vi "Grade_Saver.vi"() -> ()   [LabVIEW 2010]
panel:
  out "Letter Grade":string
  out "Final Grade":dbl
  out "Letter Grade":string
  out "Points":dbl
  in  "MP3":dbl
  out "Points":dbl
  out "Letter Grade":string
  in  "Exam":dbl
  out "Semester Grade":dbl
  out "Letter Grade":string
  out "Points":dbl
  out "Letter Grade":string
  in  "MP4":dbl
  out "Letter Grade":string
  out "Semester Grade":dbl
  out "Points":dbl
  out "Letter Grade":string
  in  "Exam":dbl
  out "Points":dbl
  out "Letter Grade":string
  in  "MP2":dbl
  out "Points":dbl
  out "Letter Grade":string
  in  "MP1":dbl
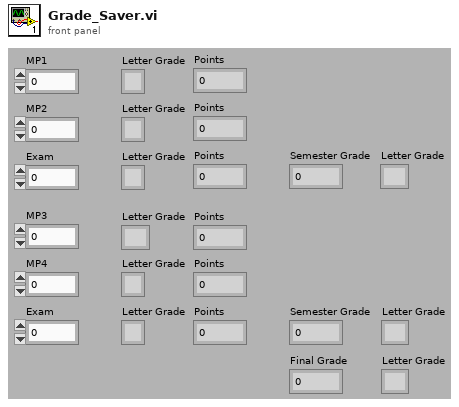
[diagram p1: front panel]
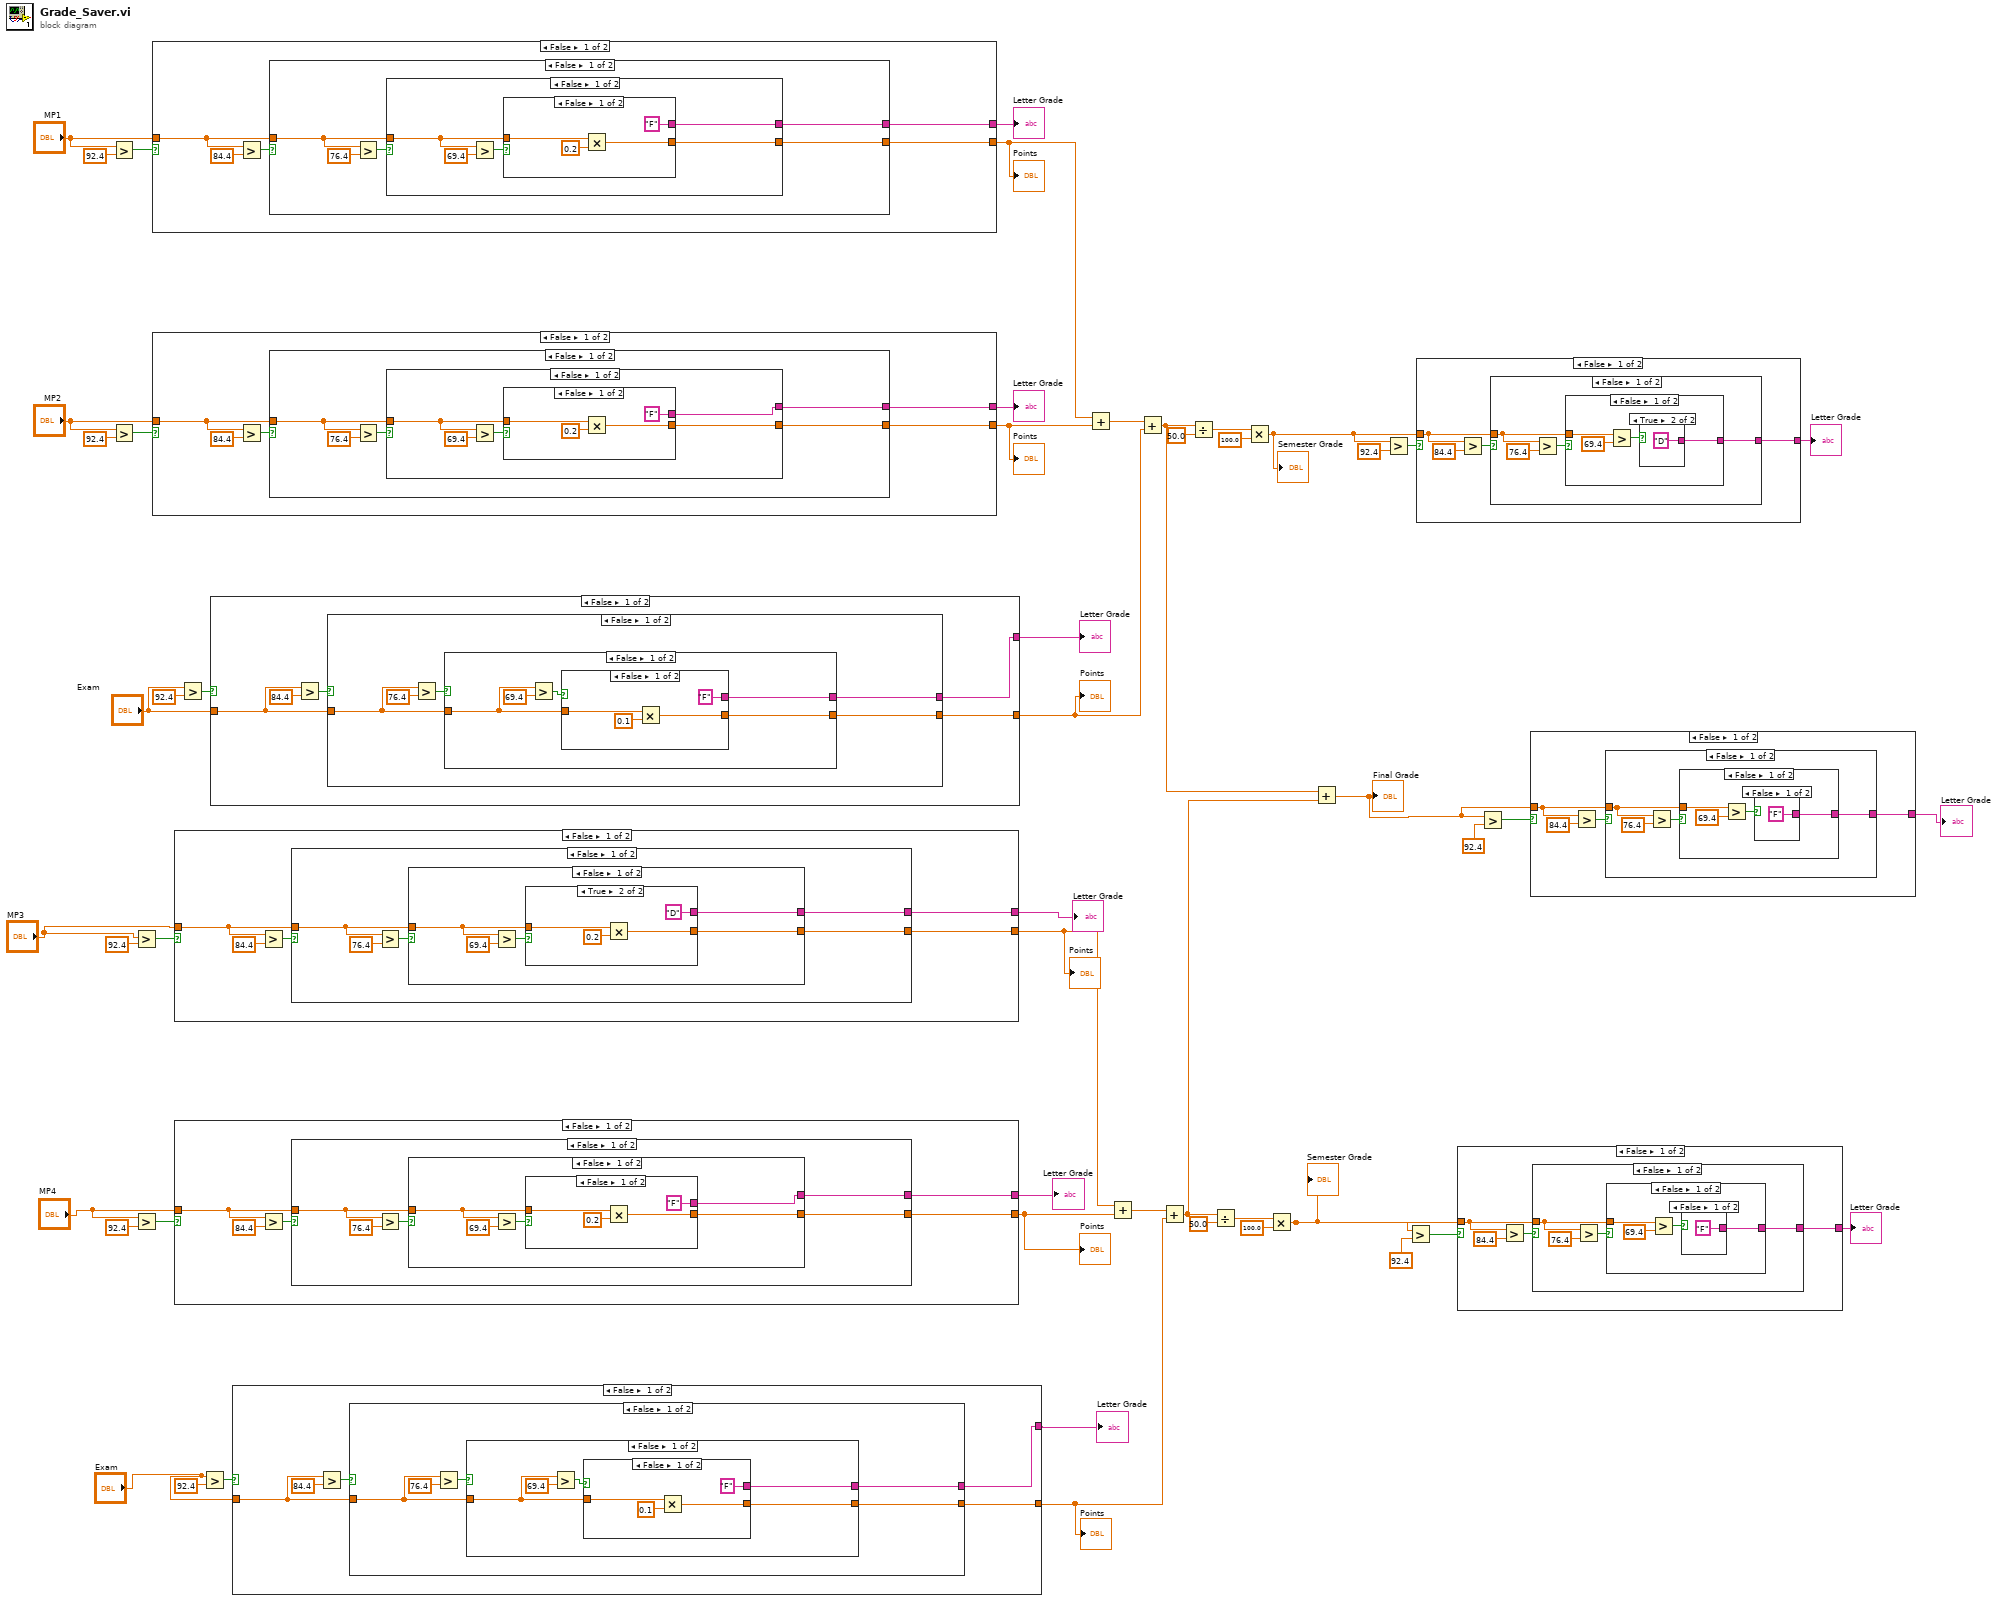
[diagram p0: block diagram]
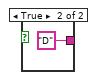
[diagram p2: hidden frame]
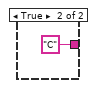
[diagram p3: hidden frame]
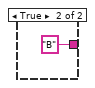
[diagram p4: hidden frame]
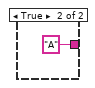
[diagram p5: hidden frame]
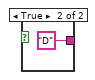
[diagram p6: hidden frame]
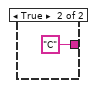
[diagram p7: hidden frame]
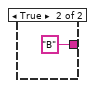
[diagram p8: hidden frame]
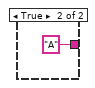
[diagram p9: hidden frame]
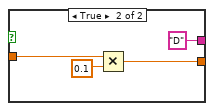
[diagram p10: hidden frame]
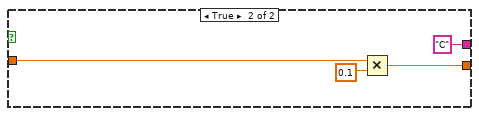
[diagram p11: hidden frame]
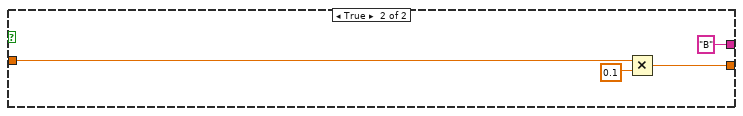
[diagram p12: hidden frame]
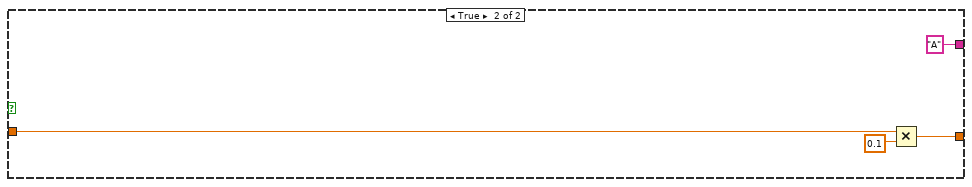
[diagram p13: hidden frame]
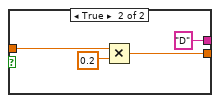
[diagram p14: hidden frame]
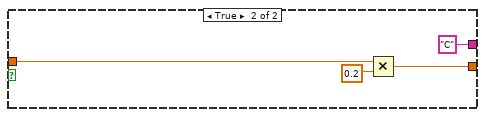
[diagram p15: hidden frame]
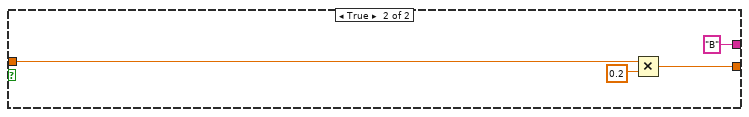
[diagram p16: hidden frame]
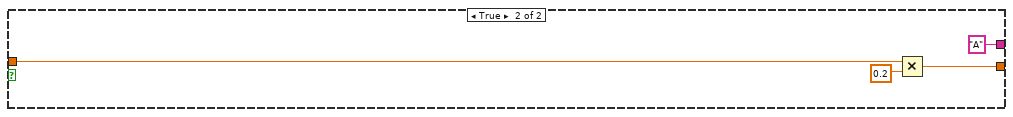
[diagram p17: hidden frame]
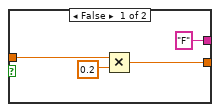
[diagram p18: hidden frame]
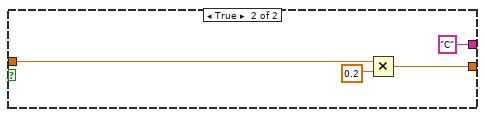
[diagram p19: hidden frame]
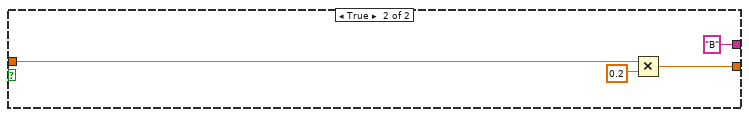
[diagram p20: hidden frame]
diagram:
  n1 = Greater?(x="MP1", y=92.4) -> (0:w51:bool)
  n2 = Greater?(x="MP2", y=92.4) -> (0:w47:bool)
  n3 = Greater?(x="MP3", y=92.4) -> (0:w28:bool)
  n4 = Greater?(x="MP4", y=92.4) -> (0:w26:bool)
  n5 = case shown="False" w51 {
    tunnel: "MP1" -> [w55 w86]
    tunnel: [w54 w85] -> w40
    tunnel: [w53 "A"] -> w49
    frame False {
      n6 = Greater?(x=w55, y=84.4) -> (0:w56:bool)
      n7 = case shown="False" w56 {
        tunnel: w55 -> [w58 w82]
        tunnel: [w59 w83] -> w54
        tunnel: [w60 "B"] -> w53
        frame False {
          n8 = Greater?(x=w58, y=76.4) -> (0:w62:bool)
          n9 = case shown="False" w62 {
            tunnel: [w65 "C"] -> w60
            tunnel: [w64 w78] -> w59
            tunnel: w58 -> [w63 w77]
            frame False {
              n10 = Greater?(x=w63, y=69.4) -> (0:w66:bool)
              n11 = case shown="False" w66 {
                tunnel: ["F" "D"] -> w65
                tunnel: [w70 w74] -> w64
                tunnel: w63 -> [w69 w73]
                frame False {
                  n12 = Multiply(x=w69, y=0.2) -> (x*y=w70:dbl)
                }
                frame True {
                  n13 = Multiply(x=w73, y=0.2) -> (x*y=w74:dbl)
                }
              }
            }
            frame True {
              n14 = Multiply(x=w77, y=0.2) -> (x*y=w78:dbl)
            }
          }
        }
        frame True {
          n15 = Multiply(x=w82, y=0.2) -> (x*y=w83:dbl)
        }
      }
    }
    frame True {
      n16 = Multiply(x=w86, y=0.2) -> (x*y=w85:dbl)
    }
  }
  "Letter Grade" <- w49
  "Points" <- w40
  n17 = case shown="False" w47 {
    tunnel: "MP2" -> [w90 w121]
    tunnel: [w89 w120] -> w39
    tunnel: [w88 "A"] -> w45
    frame False {
      n18 = Greater?(x=w90, y=84.4) -> (0:w91:bool)
      n19 = case shown="False" w91 {
        tunnel: w90 -> [w93 w117]
        tunnel: [w94 w118] -> w89
        tunnel: [w95 "B"] -> w88
        frame False {
          n20 = Greater?(x=w93, y=76.4) -> (0:w97:bool)
          n21 = case shown="False" w97 {
            tunnel: [w100 "C"] -> w95
            tunnel: [w99 w113] -> w94
            tunnel: w93 -> [w98 w112]
            frame False {
              n22 = Greater?(x=w98, y=69.4) -> (0:w101:bool)
              n23 = case shown="False" w101 {
                tunnel: ["F" "D"] -> w100
                tunnel: [w105 w109] -> w99
                tunnel: w98 -> [w104 w108]
                frame False {
                  n24 = Multiply(x=w104, y=0.2) -> (x*y=w105:dbl)
                }
                frame True {
                  n25 = Multiply(x=w108, y=0.2) -> (x*y=w109:dbl)
                }
              }
            }
            frame True {
              n26 = Multiply(x=w112, y=0.2) -> (x*y=w113:dbl)
            }
          }
        }
        frame True {
          n27 = Multiply(x=w117, y=0.2) -> (x*y=w118:dbl)
        }
      }
    }
    frame True {
      n28 = Multiply(x=w121, y=0.2) -> (x*y=w120:dbl)
    }
  }
  "Letter Grade" <- w45
  "Points" <- w39
  n29 = case shown="False" w28 {
    tunnel: "MP3" -> [w125 w156]
    tunnel: [w124 w155] -> w7
    tunnel: [w123 "A"] -> w14
    frame False {
      n30 = Greater?(x=w125, y=84.4) -> (0:w126:bool)
      n31 = case shown="False" w126 {
        tunnel: w125 -> [w128 w152]
        tunnel: [w129 w153] -> w124
        tunnel: [w130 "B"] -> w123
        frame False {
          n32 = Greater?(x=w128, y=76.4) -> (0:w132:bool)
          n33 = case shown="False" w132 {
            tunnel: [w135 "C"] -> w130
            tunnel: [w134 w148] -> w129
            tunnel: w128 -> [w133 w147]
            frame False {
              n34 = Greater?(x=w133, y=69.4) -> (0:w136:bool)
              n35 = case shown="True" w136 {
                tunnel: ["F" "D"] -> w135
                tunnel: [w140 w144] -> w134
                tunnel: w133 -> [w139 w143]
                frame False {
                  n36 = Multiply(x=w139, y=0.2) -> (x*y=w140:dbl)
                }
                frame True {
                  n37 = Multiply(x=w143, y=0.2) -> (x*y=w144:dbl)
                }
              }
            }
            frame True {
              n38 = Multiply(x=w147, y=0.2) -> (x*y=w148:dbl)
            }
          }
        }
        frame True {
          n39 = Multiply(x=w152, y=0.2) -> (x*y=w153:dbl)
        }
      }
    }
    frame True {
      n40 = Multiply(x=w156, y=0.2) -> (x*y=w155:dbl)
    }
  }
  "Letter Grade" <- w14
  "Points" <- w7
  n41 = case shown="False" w26 {
    tunnel: "MP4" -> [w160 w191]
    tunnel: [w159 w190] -> w11
    tunnel: [w158 "A"] -> w13
    frame False {
      n42 = Greater?(x=w160, y=84.4) -> (0:w161:bool)
      n43 = case shown="False" w161 {
        tunnel: w160 -> [w163 w187]
        tunnel: [w164 w188] -> w159
        tunnel: [w165 "B"] -> w158
        frame False {
          n44 = Greater?(x=w163, y=76.4) -> (0:w167:bool)
          n45 = case shown="False" w167 {
            tunnel: [w170 "C"] -> w165
            tunnel: [w169 w183] -> w164
            tunnel: w163 -> [w168 w182]
            frame False {
              n46 = Greater?(x=w168, y=69.4) -> (0:w171:bool)
              n47 = case shown="False" w171 {
                tunnel: ["F" "D"] -> w170
                tunnel: [w175 w179] -> w169
                tunnel: w168 -> [w174 w178]
                frame False {
                  n48 = Multiply(x=w174, y=0.2) -> (x*y=w175:dbl)
                }
                frame True {
                  n49 = Multiply(x=w178, y=0.2) -> (x*y=w179:dbl)
                }
              }
            }
            frame True {
              n50 = Multiply(x=w182, y=0.2) -> (x*y=w183:dbl)
            }
          }
        }
        frame True {
          n51 = Multiply(x=w187, y=0.2) -> (x*y=w188:dbl)
        }
      }
    }
    frame True {
      n52 = Multiply(x=w191, y=0.2) -> (x*y=w190:dbl)
    }
  }
  "Letter Grade" <- w13
  "Points" <- w11
  n53 = Greater?(x="Exam", y=92.4) -> (0:w43:bool)
  n54 = Greater?(x="Exam", y=92.4) -> (0:w24:bool)
  n55 = case shown="False" w43 {
    tunnel: "Exam" -> [w195 w226]
    tunnel: [w194 w225] -> w37
    tunnel: [w193 "A"] -> w41
    frame False {
      n56 = Greater?(x=w195, y=84.4) -> (0:w196:bool)
      n57 = case shown="False" w196 {
        tunnel: w195 -> [w198 w222]
        tunnel: [w199 w223] -> w194
        tunnel: [w200 "B"] -> w193
        frame False {
          n58 = Greater?(x=w198, y=76.4) -> (0:w202:bool)
          n59 = case shown="False" w202 {
            tunnel: [w205 "C"] -> w200
            tunnel: [w204 w218] -> w199
            tunnel: w198 -> [w203 w217]
            frame False {
              n60 = Greater?(x=w203, y=69.4) -> (0:w206:bool)
              n61 = case shown="False" w206 {
                tunnel: ["F" "D"] -> w205
                tunnel: [w210 w214] -> w204
                tunnel: w203 -> [w209 w213]
                frame False {
                  n62 = Multiply(x=w209, y=0.1) -> (x*y=w210:dbl)
                }
                frame True {
                  n63 = Multiply(x=w213, y=0.1) -> (x*y=w214:dbl)
                }
              }
            }
            frame True {
              n64 = Multiply(x=w217, y=0.1) -> (x*y=w218:dbl)
            }
          }
        }
        frame True {
          n65 = Multiply(x=w222, y=0.1) -> (x*y=w223:dbl)
        }
      }
    }
    frame True {
      n66 = Multiply(x=w226, y=0.1) -> (x*y=w225:dbl)
    }
  }
  "Letter Grade" <- w41
  "Points" <- w37
  n67 = case shown="False" w24 {
    tunnel: "Exam" -> [w230 w261]
    tunnel: [w229 w260] -> w10
    tunnel: [w228 "A"] -> w12
    frame False {
      n68 = Greater?(x=w230, y=84.4) -> (0:w231:bool)
      n69 = case shown="False" w231 {
        tunnel: w230 -> [w233 w257]
        tunnel: [w234 w258] -> w229
        tunnel: [w235 "B"] -> w228
        frame False {
          n70 = Greater?(x=w233, y=76.4) -> (0:w237:bool)
          n71 = case shown="False" w237 {
            tunnel: [w240 "C"] -> w235
            tunnel: [w239 w253] -> w234
            tunnel: w233 -> [w238 w252]
            frame False {
              n72 = Greater?(x=w238, y=69.4) -> (0:w241:bool)
              n73 = case shown="False" w241 {
                tunnel: ["F" "D"] -> w240
                tunnel: [w245 w249] -> w239
                tunnel: w238 -> [w244 w248]
                frame False {
                  n74 = Multiply(x=w244, y=0.1) -> (x*y=w245:dbl)
                }
                frame True {
                  n75 = Multiply(x=w248, y=0.1) -> (x*y=w249:dbl)
                }
              }
            }
            frame True {
              n76 = Multiply(x=w252, y=0.1) -> (x*y=w253:dbl)
            }
          }
        }
        frame True {
          n77 = Multiply(x=w257, y=0.1) -> (x*y=w258:dbl)
        }
      }
    }
    frame True {
      n78 = Multiply(x=w261, y=0.1) -> (x*y=w260:dbl)
    }
  }
  "Letter Grade" <- w12
  "Points" <- w10
  n79 = Add(x=w40, y=w39) -> (x+y=w38:dbl)
  n80 = Add(x=w7, y=w11) -> (x+y=w23:dbl)
  n81 = Add(x=w38, y=w37) -> (x+y=w6:dbl)
  n82 = Add(x=w23, y=w10) -> (x+y=w5:dbl)
  n83 = Divide(x=w6, y=50.0) -> (x/y=w35:dbl)
  n84 = Divide(x=w5, y=50.0) -> (x/y=w21:dbl)
  n85 = Multiply(x=w35, y=100.0) -> (x*y=w31:dbl)
  "Semester Grade" <- w31
  n86 = Multiply(x=w21, y=100.0) -> (x*y=w17:dbl)
  "Semester Grade" <- w17
  n87 = Add(x=w6, y=w5) -> (x+y=w2:dbl)
  "Final Grade" <- w2
  n88 = Greater?(x=w31, y=92.4) -> (0:w32:bool)
  n89 = Greater?(x=w17, y=92.4) -> (0:w18:bool)
  n90 = case shown="False" w32 {
    tunnel: [w264 "A"] -> w30
    tunnel: w31 -> [w263 _]
    frame False {
      n91 = Greater?(x=w263, y=84.4) -> (0:w265:bool)
      n92 = case shown="False" w265 {
        tunnel: [w268 "B"] -> w264
        tunnel: w263 -> [w267 _]
        frame False {
          n93 = Greater?(x=w267, y=76.4) -> (0:w270:bool)
          n94 = case shown="False" w270 {
            tunnel: [w272 "C"] -> w268
            tunnel: w267 -> [w271 _]
            frame False {
              n95 = Greater?(x=w271, y=69.4) -> (0:w273:bool)
              n96 = case shown="True" w273 {
                tunnel: ["F" "D"] -> w272
                frame False {
                }
                frame True {
                }
              }
            }
            frame True {
            }
          }
        }
        frame True {
        }
      }
    }
    frame True {
    }
  }
  "Letter Grade" <- w30
  n97 = case shown="False" w18 {
    tunnel: [w281 "A"] -> w9
    tunnel: w17 -> [w280 _]
    frame False {
      n98 = Greater?(x=w280, y=84.4) -> (0:w282:bool)
      n99 = case shown="False" w282 {
        tunnel: [w285 "B"] -> w281
        tunnel: w280 -> [w284 _]
        frame False {
          n100 = Greater?(x=w284, y=76.4) -> (0:w287:bool)
          n101 = case shown="False" w287 {
            tunnel: [w289 "C"] -> w285
            tunnel: w284 -> [w288 _]
            frame False {
              n102 = Greater?(x=w288, y=69.4) -> (0:w290:bool)
              n103 = case shown="False" w290 {
                tunnel: ["F" "D"] -> w289
                frame False {
                }
                frame True {
                }
              }
            }
            frame True {
            }
          }
        }
        frame True {
        }
      }
    }
    frame True {
    }
  }
  "Letter Grade" <- w9
  n104 = Greater?(x=w2, y=92.4) -> (0:w3:bool)
  n105 = case shown="False" w3 {
    tunnel: [w298 "A"] -> w1
    tunnel: w2 -> [w297 _]
    frame False {
      n106 = Greater?(x=w297, y=84.4) -> (0:w299:bool)
      n107 = case shown="False" w299 {
        tunnel: [w302 "B"] -> w298
        tunnel: w297 -> [w301 _]
        frame False {
          n108 = Greater?(x=w301, y=76.4) -> (0:w304:bool)
          n109 = case shown="False" w304 {
            tunnel: [w306 "C"] -> w302
            tunnel: w301 -> [w305 _]
            frame False {
              n110 = Greater?(x=w305, y=69.4) -> (0:w307:bool)
              n111 = case shown="False" w307 {
                tunnel: ["F" "D"] -> w306
                frame False {
                }
                frame True {
                }
              }
            }
            frame True {
            }
          }
        }
        frame True {
        }
      }
    }
    frame True {
    }
  }
  "Letter Grade" <- w1
